vi "Init.vi"(8 "error in (no error)":errorcluster) -> (0 "error out":errorcluster, 3 "InfoService out":refnum<class "NodeStatus.lvclass">)   [LabVIEW 2020, in "Vecto.lvlib" / "NodeStatus.lvclass"]
uses:
  NodeStatus.lvclass
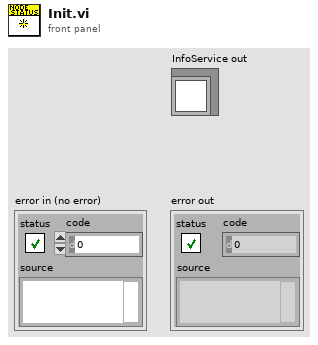
[diagram p1: front panel]
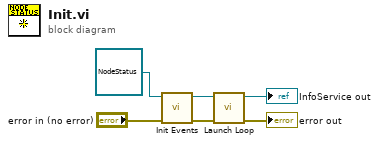
[diagram p0: block diagram]
diagram:
  n1 = call "Init Events.vi"("error in (no error)"="error in (no error)", "InfoService in"=refnum<class "NodeStatus.lvclass"> refnum) -> ("error out"=w5:errorcluster, "InfoService out"=w2:refnum<class "NodeStatus.lvclass">)  [unwired: 8 in]
  n2 = call "Launch Loop.vi"("error in (no error)"=w5, "InfoService in"=w2) -> ("error out"=→"error out":errorcluster, "InfoService out"=→"InfoService out":refnum<class "NodeStatus.lvclass">)  [unwired: 8 in]
